vi "Read ADU Packet.vi"(8 "error in":errorcluster, 10 "protocol layer":refnum<class "Network Protocol.lvclass">, 11 "RTU transmission data unit in":refnum<class "RTU Data Unit.lvclass">) -> (0 "error out":errorcluster, 1 "modbus data unit":refnum<class "Modbus Data Unit.lvclass">, 2 "protocol layer out":refnum<class "Network Protocol.lvclass">, 3 "RTU transmission data unit out":refnum<class "RTU Data Unit.lvclass">, 5 "PDU Valid?":bool)   [LabVIEW 2012, in "RTU Data Unit.lvclass"]
doc: "This uses the protocol layer to read a modbus packet off of the bus, wrapped in the RTU transmission data unit."
uses:
  RTU Data Unit.lvclass
  Modbus Data Unit/Modbus Data Unit.lvclass
  Network Protocol/Network Protocol.lvclass
  Network Protocol/Network Master/Serial/Serial Master.lvclass
  Network Protocol/Network Slave/Serial/Serial Slave.lvclass
  Network Protocol/Network Master/Serial/Serial Master.lvclass/Serial Master.ctl
  Network Protocol/Network Slave/Serial/Serial Slave.lvclass/Serial Slave.ctl
  RTU Data Unit.lvclass/RTU Data Unit.ctl
  Transmission Data Unit.lvclass/Transmission Data Unit.ctl
  Serial Interface/Serial Data Unit.lvclass/Serial Data Unit.ctl
  Modbus Data Unit/Modbus Data Unit.lvclass/Modbus Data Unit.ctl
  Serial Interface/Serial acquisition states.ctl
  buffer element.ctl
  <vilib>/ErrorRing/Error Ring.xnode
  Serial Interface/Serial Data Unit.lvclass
  Transmission Data Unit.lvclass
  Network Protocol/Serial Shared Components/Serial Shared Components.lvlib
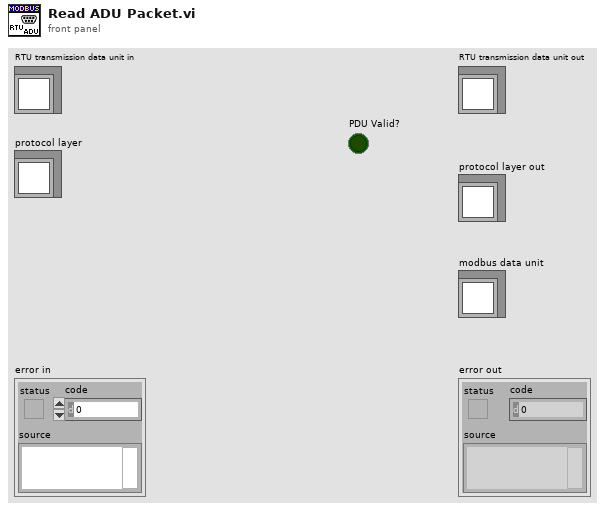
[diagram p1: front panel]
types:
  T1 = typedef "RTU Data Unit.lvclass/buffer element.ctl" = cluster{"data":u8[], "packets contained":i32}
  T2 = typedef "Serial Data Unit.lvclass/Serial acquisition states.ctl" = enum16{"Wait for frame", "Check for validity"}
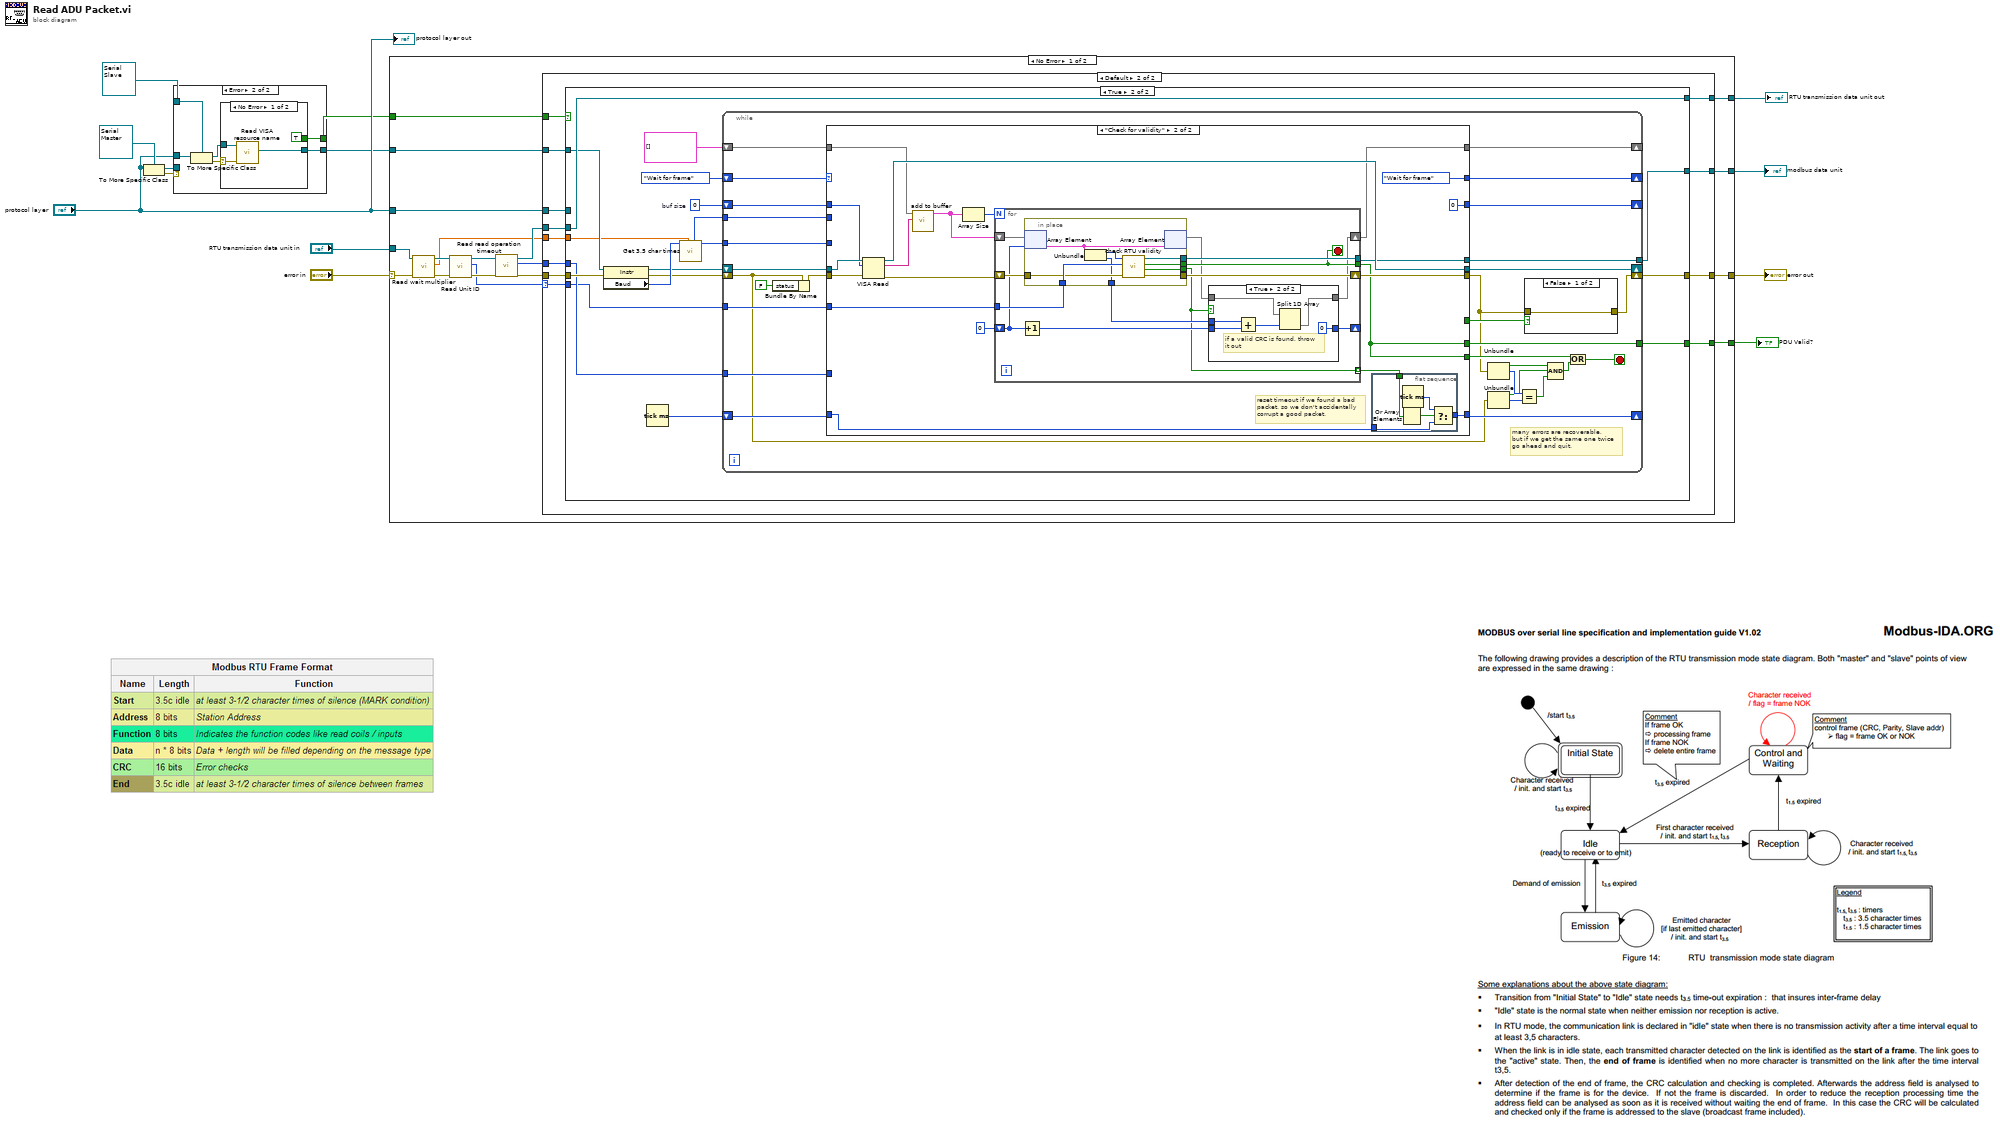
[diagram p0: block diagram]
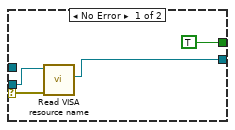
[diagram p2: hidden frame]
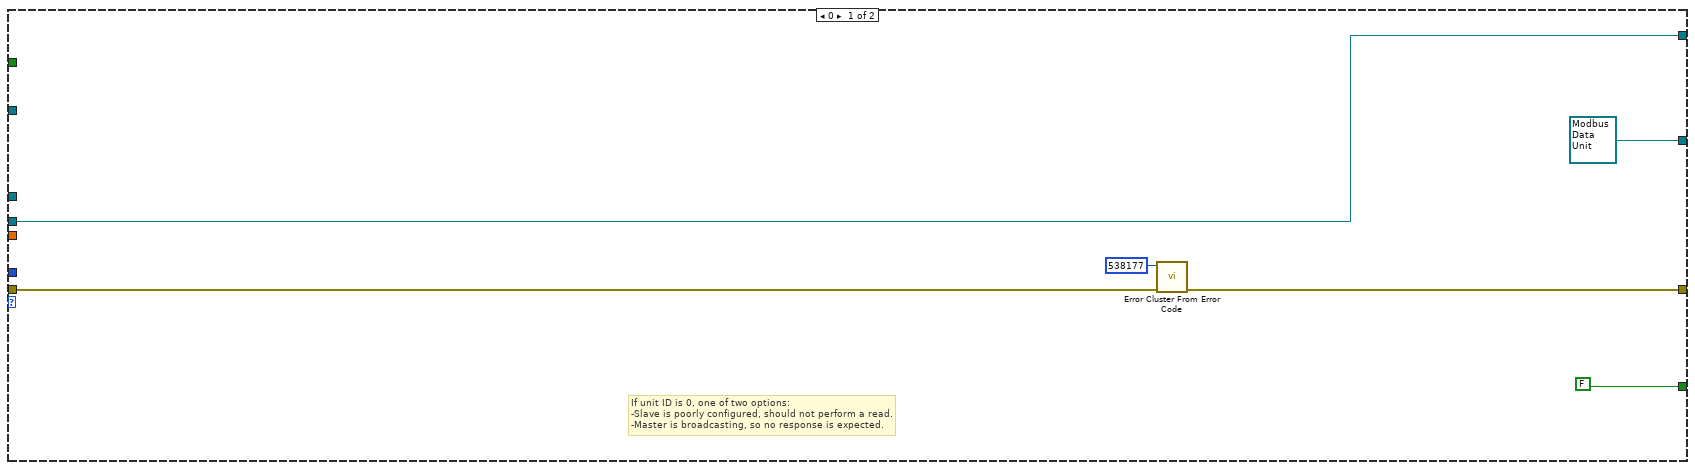
[diagram p4: hidden frame]
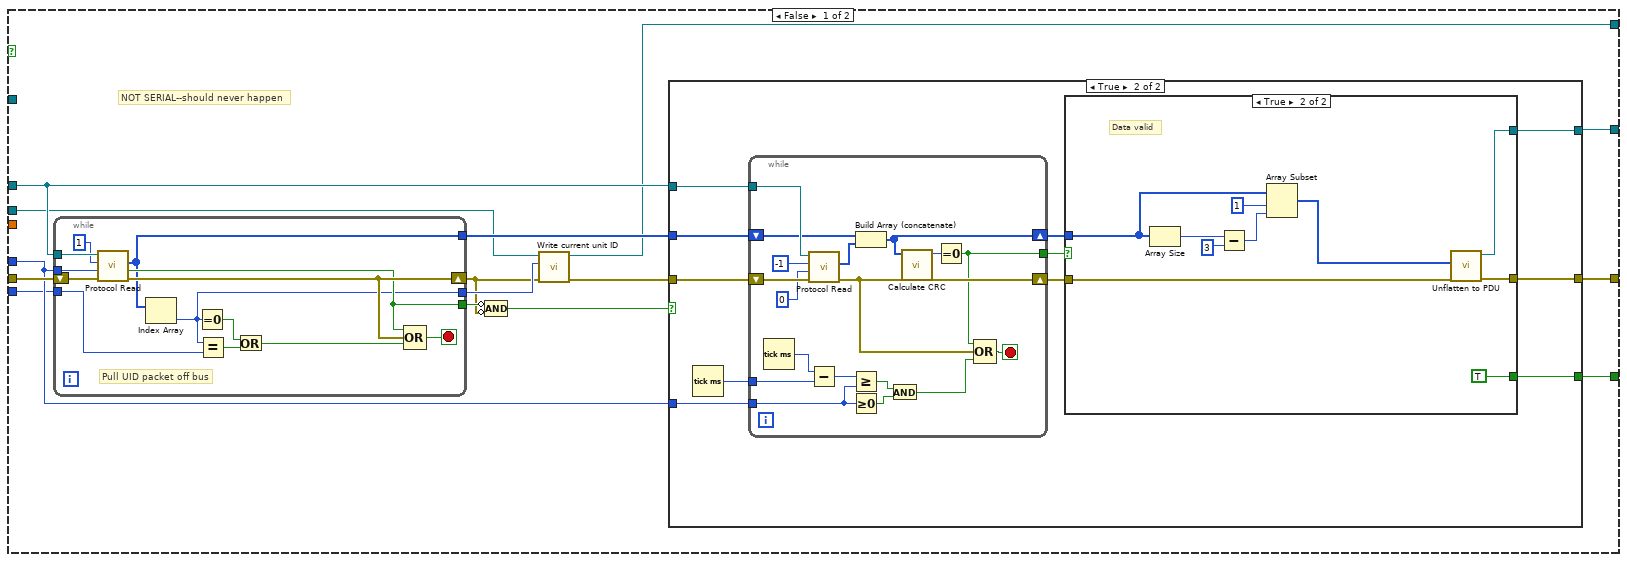
[diagram p5: hidden frame]
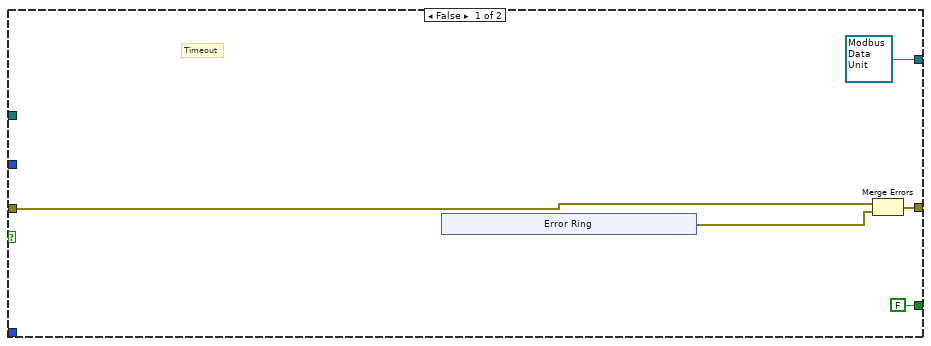
[diagram p6: hidden frame]
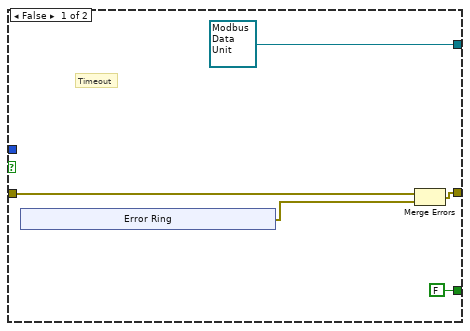
[diagram p7: hidden frame]
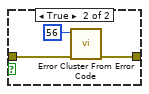
[diagram p8: hidden frame]
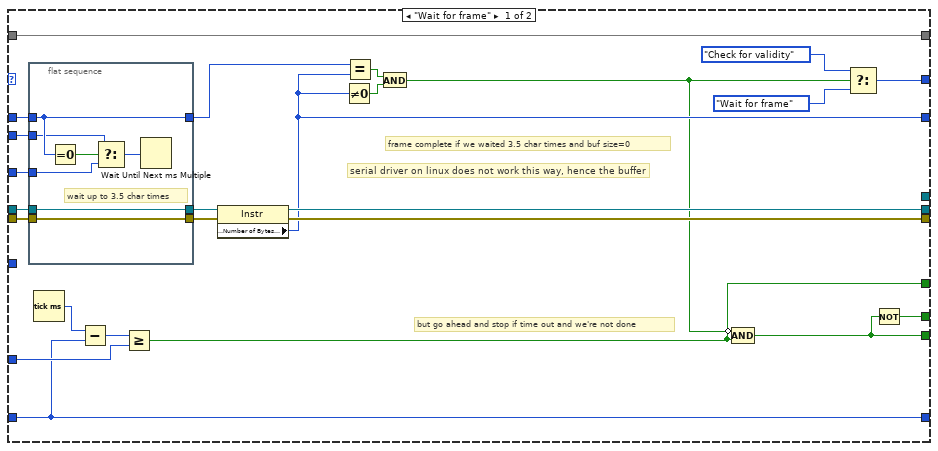
[diagram p9: hidden frame]
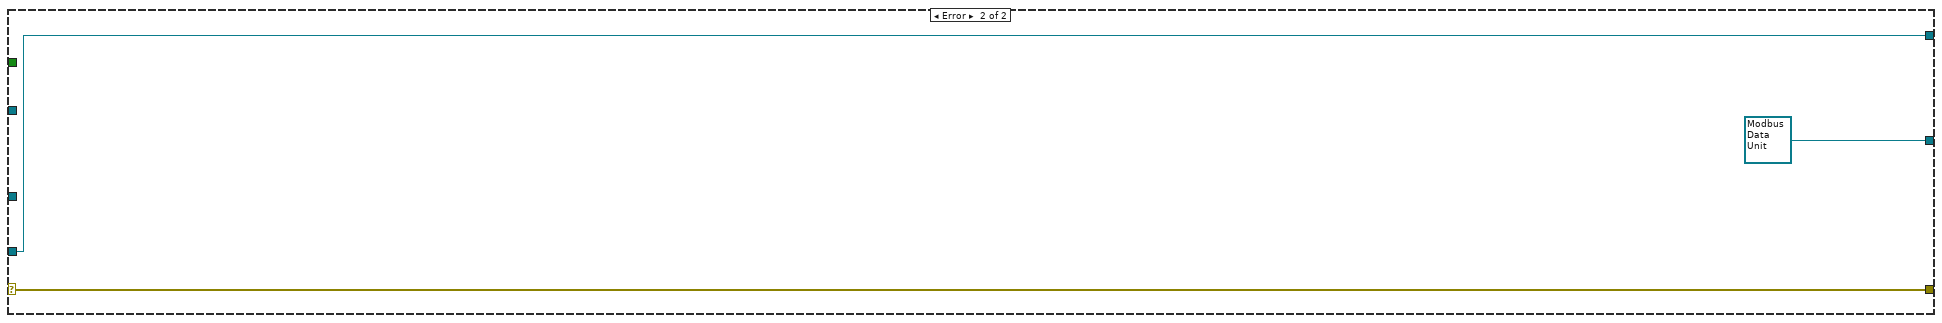
[diagram p11: hidden frame]
diagram:
  n1 = To More Specific Class(target class=refnum<class "Serial Master.lvclass"> refnum ("Serial Master"), reference="protocol layer") -> (specific class reference=w2:refnum<class "Serial Master.lvclass">, error out=w6:errorcluster)  [unwired: 1 in]
  n2 = case shown="Error" w6 {
    selector: w6 -> [w16 _]
    tunnel: "protocol layer" -> [_ w23]
    tunnel: [TRUE w21] -> w4
    tunnel: refnum<class "Serial Slave.lvclass"> refnum ("Serial Slave") -> [_ w20]
    tunnel: [w14 w18] -> w1
    tunnel: w2 -> [w15 _]
    frame No Error {
      n3 = call "Read VISA resource name.vi"("error in (no error)"=w16, "Serial Master in"=w15) -> ("VISA resource name"=w14:refnum<visa-resource-name>)  [unwired: 7 in, 2 out]
    }
    frame Error {
      n4 = To More Specific Class(target class=w20, reference=w23) -> (specific class reference=w19:refnum<class "Serial Slave.lvclass">, error out=w22:errorcluster)  [unwired: 1 in]
      n5 = case shown="No Error" w22 {
        selector: w22 -> [w26 _]
        tunnel: [TRUE _] -> w21
        tunnel: w19 -> [w25 _]
        tunnel: [w24 _] -> w18
        frame No Error {
          n6 = call "Read VISA resource name.vi"("error in (no error)"=w26, "Serial Slave in"=w25) -> ("VISA resource name"=w24:refnum<visa-resource-name>)  [unwired: 7 in, 2 out]
        }
        frame Error {
        }
      }
    }
  }
  n7 = case shown="No Error" "error in" {
    selector: "error in" -> [w31 w290]
    tunnel: [w45 w290] -> w12
    tunnel: "RTU transmission data unit in" -> [w32 w288]
    tunnel: "protocol layer" -> [w43 _]
    tunnel: [w44 refnum<class "Modbus Data Unit.lvclass"> refnum ("modbus data unit")] -> w11
    tunnel: [w42 w288] -> w9
    tunnel: [w35 _] -> w8
    tunnel: w4 -> [w34 _]
    tunnel: w1 -> [w33 _]
    frame No Error {
      n8 = call "Read wait multiplier.vi"("error in (no error)"=w31, "RTU Data Unit in"=w32) -> ("error out"=w30:errorcluster, "wait multiplier"=w28:sgl, "RTU Data Unit out"=w29:refnum<class "RTU Data Unit.lvclass">)  [unwired: 7 in]
      n9 = call "Read Unit ID.vi"("error in"=w30, "transmission data unit in"=w29) -> ("error out"=w39:errorcluster, "unit ID"=w37:u8, "transmission data unit out"=w38:refnum<class "RTU Data Unit.lvclass">)  [unwired: 7 in]
      n10 = call "Read read operation timeout.vi"("error in (no error)"=w39, "transmission data unit in"=w38) -> ("error out"=w40:errorcluster, "read operation timeout"=w36:i32, "transmission data unit out"=w41:refnum<class "RTU Data Unit.lvclass">)  [unwired: 7 in]
      n11 = case shown="Default" w37 {
        selector: w37 -> [_ w58]
        tunnel: w40 -> [w51 w63]
        tunnel: [w47 w62] -> w45
        tunnel: [refnum<class "Modbus Data Unit.lvclass"> refnum ("modbus data unit out") w61] -> w44
        tunnel: w43 -> [_ w60]
        tunnel: w36 -> [_ w59]
        tunnel: w41 -> [w50 w56]
        tunnel: [w50 w57] -> w42
        tunnel: [FALSE w55] -> w35
        tunnel: w34 -> [_ w54]
        tunnel: w33 -> [_ w53]
        tunnel: w28 -> [_ w52]
        frame 0 {
          # "If unit ID is 0, one of two options:\n-Slave is poorly configured, should not perform a read.\n-Master is broadcasting, so no response is expected."
          n12 = call <vilib>:"Error Cluster From Error Code.vi"("error in (no error)"=w51, "error code (0)"=538177) -> ("error out"=w47:errorcluster)  [unwired: 7 in]
        }
        frame Default {
          n13 = case shown="True" w54 {
            tunnel: w63 -> [w78 w164]
            tunnel: [w75 w161] -> w62
            tunnel: [w74 w152] -> w61
            tunnel: w60 -> [w73 _]
            tunnel: w59 -> [w71 w156]
            tunnel: w58 -> [w70 w153]
            tunnel: [w69 w166] -> w57
            tunnel: w56 -> [w67 w166]
            tunnel: [w64 w154] -> w55
            tunnel: w53 -> [_ w163]
            tunnel: w52 -> [_ w149]
            frame False {
              # "NOT SERIAL--should never happen"
              n14 = while {
                shift-right: [w145] -> w65
                shift-left: w78 -> [w148]
                tunnel: w71 -> [w143]
                tunnel: w70 -> [w139]
                tunnel: [w138] -> w77
                tunnel: [w137] -> w72
                tunnel: w73 -> [w147]
                tunnel: [w136] -> w66
                stop <- w146 stop-if-true
                # "Pull UID packet off bus"
                n15 = call-dynamic "Protocol Read.vi"("error in"=w148, "timeout"=w143, "bytes to read"=1, "protocol layer in"=w147) -> ("error out"=w145:errorcluster, "timed out?"=w138:bool, "data"=w137:u8[])  [unwired: 4 in, 1 out]
                n16 = Index Array(array=w137) -> (element=w136:u8)  [unwired: 1 in]
                n17 = Equal To 0?(x=w136) -> (x = 0?=w140:bool)
                n18 = Equal?(x=w136, y=w139) -> (x = y?=w142:bool)
                n19 = Or(x=w140, y=w142) -> (x .or. y?=w141:bool)
                n20 = Compound Arithmetic op=OR(w138, w145, w141) -> (w146:bool)
              }
              n21 = Compound Arithmetic op=AND(invert w77, invert w65) -> (w76:bool)
              n22 = call "Write current unit ID.vi"("error in (no error)"=w65, "request unit ID"=w66, "Serial Data Unit in"=w67) -> ("error out"=w68:errorcluster, "Serial Data Unit out"=w69:refnum<class "RTU Data Unit.lvclass">)  [unwired: 7 in]
              n23 = case shown="True" w76 {
                tunnel: w68 -> [w81 w98]
                tunnel: [w82 w90] -> w75
                tunnel: [refnum<class "Modbus Data Unit.lvclass"> refnum ("modbus data unit out") w91] -> w74
                tunnel: w73 -> [_ w94]
                tunnel: w72 -> [_ w95]
                tunnel: w71 -> [_ w96]
                tunnel: [FALSE w88] -> w64
                frame False {
                  # "Timeout"
                  n24 = xnode "Error Ring"() -> ("error out"=w83:errorcluster)
                  n25 = Merge Errors(w81, w83) -> (w82:errorcluster)
                }
                frame True {
                  n26 = Tick Count (ms)() -> (millisecond timer value=w97:u32)
                  n27 = while {
                    shift-right: [w121] -> w92
                    shift-left: w98 -> [w127]
                    tunnel: w97 -> [w135]
                    tunnel: w96 -> [w132]
                    shift-right: [w119] -> w89
                    shift-left: w95 -> [w123]
                    tunnel: w94 -> [w126]
                    tunnel: [w118] -> w93
                    stop <- w129 stop-if-true
                    n28 = Tick Count (ms)() -> (millisecond timer value=w134:u32)
                    n29 = call-dynamic "Protocol Read.vi"("error in"=w127, "timeout"=0, "bytes to read"=-1, "protocol layer in"=w126) -> ("error out"=w121:errorcluster, "data"=w122:u8[])  [unwired: 4 in, 2 out]
                    n30 = Subtract(x=w134, y=w135) -> (x-y=w133:u32)
                    n31 = Greater Or Equal?(x=w133, y=w132) -> (x >= y?=w130:bool)
                    n32 = Greater Or Equal To 0?(x=w132) -> (x >= 0?=w131:bool)
                    n33 = Build Array (concatenate)(w123, w122) -> (w119:u8[])
                    n34 = And(x=w130, y=w131) -> (x .and. y?=w128:bool)
                    n35 = call "Calculate CRC.vi"("data"=w119) -> ("CRC-16"=w120:u16)  [unwired: 10 in]
                    n36 = Equal To 0?(x=w120) -> (x = 0?=w118:bool)
                    n37 = Compound Arithmetic op=OR(w118, w121, w128) -> (w129:bool)
                  }
                  n38 = case shown="True" w93 {
                    tunnel: w92 -> [w101 w115]
                    tunnel: [refnum<class "Modbus Data Unit.lvclass"> refnum ("modbus data unit") w116] -> w91
                    tunnel: [w100 w117] -> w90
                    tunnel: w89 -> [_ w109]
                    tunnel: [FALSE TRUE] -> w88
                    frame False {
                      # "Timeout"
                      n39 = xnode "Error Ring"() -> ("error out"=w102:errorcluster)
                      n40 = Merge Errors(w101, w102) -> (w100:errorcluster)
                    }
                    frame True {
                      # "Data valid"
                      n41 = Array Size(array=w109) -> (size(s)=w113:i32)
                      n42 = Subtract(x=w113, y=3) -> (x-y=w111:i32)
                      n43 = Array Subset(array=w109, index=1, length=w111) -> (w110:u8[])
                      n44 = call "Unflatten to PDU.vi"("error in"=w115, "modbus data unit data"=w110) -> ("error out"=w117:errorcluster, "modbus data unit out"=w116:refnum<class "Modbus Data Unit.lvclass">)  [unwired: 8 in]
                    }
                  }
                }
              }
            }
            frame True {
              w158 = u32 0  # buf size
              n45 = property class="Instr"(reference=w163, error in=w164) -> (reference out=w160:refnum<visa-resource-name>, error out=w162:errorcluster, "Baud"=w165:u32)
              n46 = Tick Count (ms)() -> (millisecond timer value=w157:u32)
              n47 = call "Get 3.5 char times.vi"("wait multiplier"=w149, "baud rate"=w165) -> ("wait time (ms)"=w155:u32, "initial wait (ms)"=w151:u32)  [unwired: 8 in]
              n48 = while {
                shift-right: [w183] -> w161
                shift-left: w162 -> [w173]
                shift-right: [w189] -> _
                shift-left: w160 -> [w195]
                shift-right: [w188] -> _
                shift-left: Serial_acquisition_states."Wait for frame" ("Serial Acquisition States") -> [w196]
                shift-right: [w190] -> _
                shift-left: w158 -> [w192]
                tunnel: w156 -> [w193]
                tunnel: w155 -> [w191]
                tunnel: [w187] -> w154
                tunnel: w153 -> [w186]
                tunnel: [w185] -> w152
                tunnel: w151 -> [w182]
                shift-right: [w180] -> _
                shift-left: T1[] [] -> [w181]
                shift-right: [w179] -> _
                shift-left: w157 -> [w194]
                stop <- w176 stop-if-true
                # "many errors are recoverable,\nbut if we get the same one twice\ngo ahead and quit."
                n49 = Bundle By Name(cluster=w173, "status"=FALSE) -> (w178:errorcluster)
                n50 = case shown="\"Check for validity\"" w196 {
                  tunnel: w195 -> [w221 w251]
                  tunnel: w178 -> [w220 w252]
                  tunnel: w194 -> [w201 w234]
                  tunnel: w193 -> [w223 _]
                  tunnel: w192 -> [w218 w250]
                  tunnel: w191 -> [w217 _]
                  tunnel: [w208 u32 0 ("Bytes at Port")] -> w190
                  tunnel: [w205 w235] -> w175
                  tunnel: [w213 w245] -> w174
                  tunnel: [w212 w244] -> w189
                  tunnel: [w209 Serial_acquisition_states."Wait for frame" ("Serial Acquisition States")] -> w188
                  tunnel: [w206 w235] -> w187
                  tunnel: w186 -> [_ w248]
                  tunnel: [_ w242] -> w185
                  tunnel: [w204 _] -> w184
                  tunnel: w182 -> [w203 _]
                  tunnel: w181 -> [w202 w241]
                  tunnel: [w202 w237] -> w180
                  tunnel: [w201 w236] -> w179
                  frame "Wait for frame" {
                    # "serial driver on linux does not work this way, hence the buffer"
                    # "but go ahead and stop if time out and we're not done"
                    # "frame complete if we waited 3.5 char times and buf size=0"
                    n51 = flat-sequence {
                      tunnel: [w232] -> w222
                      tunnel: w221 -> [w232]
                      tunnel: w220 -> [w231]
                      tunnel: [w231] -> w219
                      tunnel: w218 -> [w230]
                      tunnel: [w230] -> w214
                      tunnel: w217 -> [w228]
                      tunnel: w203 -> [w226]
                      frame #0 {
                        # "wait up to 3.5 char times"
                        n52 = Equal To 0?(x=w230) -> (x = 0?=w229:bool)
                        n53 = Select(t=w226, s=w229, f=w228) -> (s? t:f=w227:u32)
                        n54 = Wait Until Next ms Multiple(millisecond multiple=w227) -> ()  [unwired: 1 out]
                      }
                    }
                    n55 = Tick Count (ms)() -> (millisecond timer value=w225:u32)
                    n56 = Subtract(x=w225, y=w201) -> (x-y=w224:u32)
                    n57 = Greater Or Equal?(x=w224, y=w223) -> (x >= y?=w204:bool)
                    n58 = property class="Instr"(reference=w222, error in=w219) -> (reference out=w212:refnum<visa-resource-name>, error out=w213:errorcluster, "Serial Settings:Number of Bytes at Serial Port"=w208:u32)
                    n59 = Not Equal To 0?(x=w208) -> (x != 0?=w216:bool)
                    n60 = Equal?(x=w214, y=w208) -> (x = y?=w215:bool)
                    n61 = And(x=w215, y=w216) -> (x .and. y?=w207:bool)
                    n62 = Compound Arithmetic op=AND(invert w207, w204) -> (w205:bool)
                    n63 = Select(t=Serial_acquisition_states."Check for validity" ("Serial Acquisition States"), s=w207, f=Serial_acquisition_states."Wait for frame" ("Serial Acquisition States")) -> (s? t:f=w209:T2)
                    n64 = Not(x=w205) -> (.not. x?=w206:bool)
                  }
                  frame "Check for validity" {
                    # "reset timeout if we found a bad\npacket, so we don't accidentally\ncorrupt a good packet."
                    n65 = VISA Read(VISA resource name=w251, byte count=w250, error in (no error)=w252) -> (VISA resource name out=w244:refnum<visa-resource-name>, read buffer=w249:string, error out=w247:errorcluster)  [unwired: 1 out]
                    n66 = call "add to buffer.vi"("read data"=w249, "buffer in"=w241) -> ("buffer out"=w238:T1[])  [unwired: 9 in]
                    n67 = Array Size(array=w238) -> (size(s)=w239:i32)
                    n68 = for {
                      N: w239 -> [_]
                      tunnel: w248 -> [w265]
                      tunnel: [w268] -> w242
                      shift-right: [w269] -> w245
                      shift-left: w247 -> [w270]
                      shift-right: [w260] -> _
                      shift-left: 0 -> [w264]
                      shift-right: [w261] -> w237
                      shift-left: w238 -> [w266]
                      tunnel: [w267] -> w235
                      tunnel: [w258] -> w233 mode=indexing
                      stop <- w267 stop-if-true
                      n69 = Increment(x=w264) -> (x+1=w263:i32)
                      n70 = in-place {
                        in-place-border: w265 -> [w287]
                        in-place-border: w270 -> [w286]
                        in-place-border: [w285] -> w269
                        in-place-border: [w284] -> w268
                        in-place-border: [w283] -> w267
                        in-place-border: [w282] -> w258
                        in-place-border: [w279] -> w259
                        n71 = in-place-array #1(w266, w264) -> (w281:T1)
                        n72 = Unbundle(w281) -> ("data"=w280:u8[], "packets contained"=w279:i32)
                        n73 = call "check RTU validity.vi"("error in (no error)"=w286, "unit ID"=w287, "unsigned byte array"=w280) -> ("error out"=w285:errorcluster, "valid packet"=w282:bool, "valid PDU"=w283:bool, "Modbus Data Unit out"=w284:refnum<class "Modbus Data Unit.lvclass">)  [unwired: 5 in]
                        n74 = in-place-array #1(w281) -> (w262:T1[])  [unwired: 1 out]
                      }
                      n75 = case shown="True" w258 {
                        tunnel: w262 -> [w272 w278]
                        tunnel: w263 -> [w271 w277]
                        tunnel: [w272 w275] -> w261
                        tunnel: [w271 0] -> w260
                        tunnel: w259 -> [_ w273]
                        frame False {
                        }
                        frame True {
                          # "if a valid CRC is found, throw\nit out"
                          n76 = Add(x=w273, y=w277) -> (x+y=w274:i32)
                          n77 = Split 1D Array(array=w278, index=w274) -> (second subarray=w275:T1[])  [unwired: 1 out]
                        }
                      }
                    }
                    n78 = flat-sequence {
                      tunnel: [w257] -> w236
                      tunnel: w234 -> [w256]
                      tunnel: w233 -> [w254]
                      frame #0 {
                        n79 = Or Array Elements(Boolean array=w254) -> (logical OR=w255:bool)
                        n80 = Tick Count (ms)() -> (millisecond timer value=w253:u32)
                        n81 = Select(t=w253, s=w255, f=w256) -> (s? t:f=w257:u32)
                      }
                    }
                  }
                }
                n82 = Unbundle(w174) -> ("status"=w170:bool, "code"=w171:i32)  [unwired: 1 out]
                n83 = Unbundle(w173) -> ("status"=w169:bool, "code"=w172:i32)  [unwired: 1 out]
                n84 = Equal?(x=w171, y=w172) -> (x = y?=w167:bool)
                n85 = case shown="False" w184 {
                  tunnel: w174 -> [w197 w200]
                  tunnel: [w197 w199] -> w183
                  frame False {
                  }
                  frame True {
                    n86 = call <vilib>:"Error Cluster From Error Code.vi"("error in (no error)"=w200, "error code (0)"=56) -> ("error out"=w199:errorcluster)  [unwired: 7 in]
                  }
                }
                n87 = Compound Arithmetic op=AND(w170, w169, w167) -> (w168:bool)
                n88 = Or(x=w175, y=w168) -> (x .or. y?=w176:bool)
              }
            }
          }
        }
      }
    }
    frame Error {
    }
  }
  "RTU transmission data unit out" <- w9
  "modbus data unit" <- w11
  "error out" <- w12
  "PDU Valid?" <- w8
  "protocol layer out" <- "protocol layer"
